vi "svx_Oct_Waterfall XYZ Scale.vi"(8 "Minimum":dbl, 9 "Maximum":dbl, 10 "Offset":dbl, 11 "Multiplier":dbl) -> (0 "Scaled.Minimum":dbl, 1 "Scaled.Maximum":dbl, 2 "Range.Minimum":dbl, 3 "Range.Maximum":dbl, 5 "flipped?":bool)   [LabVIEW 2017, in "SVX Octave Waterfall Graph.xctl"]
uses:
  <vilib>/addons/_XControls/Octave Waterfall Graph/SVX Octave Waterfall Graph.xctl
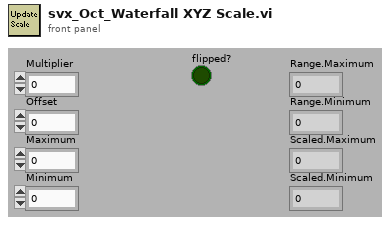
[diagram p1: front panel]
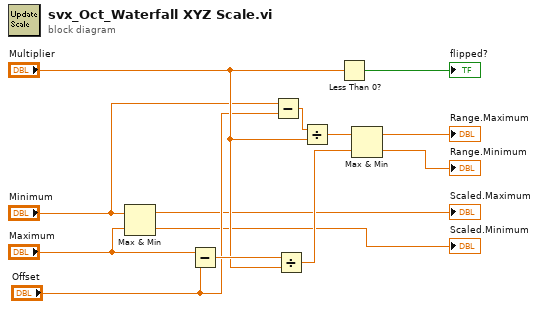
[diagram p0: block diagram]
diagram:
  n1 = Max & Min(x="Minimum", y="Maximum") -> (max(x,y)=→"Scaled.Maximum":dbl, min(x,y)=→"Scaled.Minimum":dbl)
  n2 = Subtract(x="Maximum", y="Offset") -> (x-y=w10:dbl)
  n3 = Subtract(x="Minimum", y="Offset") -> (x-y=w13:dbl)
  n4 = Divide(x=w10, y="Multiplier") -> (x/y=w11:dbl)
  n5 = Divide(x=w13, y="Multiplier") -> (x/y=w12:dbl)
  n6 = Less Than 0?(x="Multiplier") -> (x < 0?=→"flipped?":bool)
  n7 = Max & Min(x=w12, y=w11) -> (max(x,y)=→"Range.Maximum":dbl, min(x,y)=→"Range.Minimum":dbl)
